vi "New from extension bytes.vi"(9 "Ext size":T1, 10 "Payload bytes":u8[](array[numeric]), 11 "Payload Ext Type":i8) -> (0 "error out":errorcluster, 3 "MsgPackExt out":refnum<class "MsgPackExt.lvclass">)   [LabVIEW 2020, in "MessagePack.lvlib" / "MsgPackExt.lvclass"]
uses:
  MsgPackExt.lvclass
  Requested ext size.ctl
  Typedefs/MsgPack Object Types.ctl
  MsgPackExt.lvclass/MsgPackExt.ctl
  MessagePack.lvlib
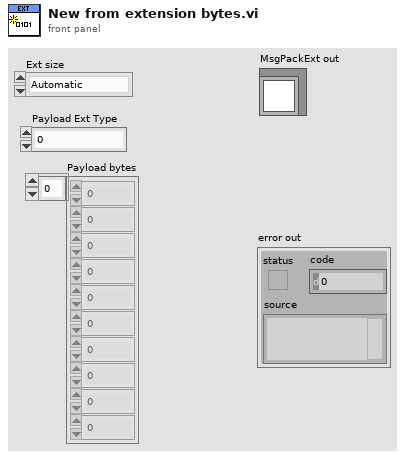
[diagram p1: front panel]
types:
  T1 = typedef "MessagePack.lvlib/MsgPackExt.lvclass/Requested ext size.ctl" = enum16{"Automatic", "Fixed 1-byte", "Fixed 2-bytes", "Fixed 4-bytes", "Fixed 8-bytes", "Fixed 16-bytes", "Up to 8 bytes", "Up to 16 bytes", "Up to 32 bytes"}
  T2 = typedef "MessagePack.lvlib/MsgPack Object Types.ctl" = enum16{"UNSUPPORTED", "POSINT", "NEGINT", "FIXMAP", "FIXARRAY", "FIXSTR", "NIL", "FALSE", "TRUE", "BIN8", "BIN16", "BIN32", "EXT8", "EXT16", "EXT32", "FLOAT32", "FLOAT64", "UINT8", "UINT16", "UINT32", "UINT64", "INT8", "INT16", "INT32", "INT64", "FIXEXT1", "FIXEXT2", "FIXEXT4", "FIXEXT8", "FIXEXT16", "STR8", "STR16", "STR32", "ARRAY16", "ARRAY32", "MAP16", "MAP32"}
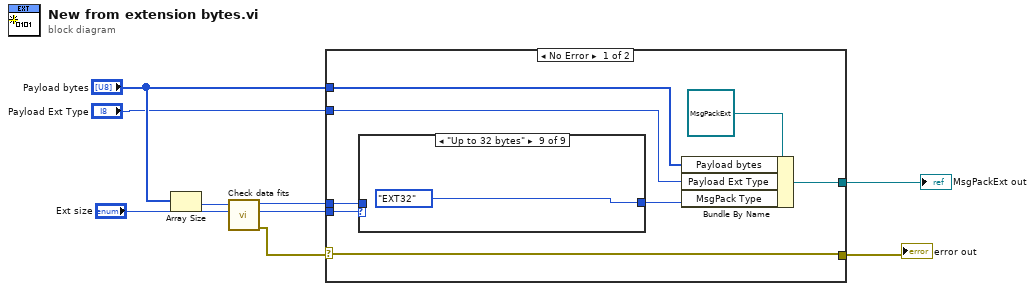
[diagram p0: block diagram]
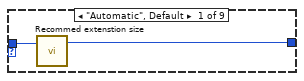
[diagram p2: hidden frame]
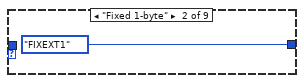
[diagram p3: hidden frame]
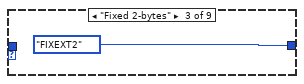
[diagram p4: hidden frame]
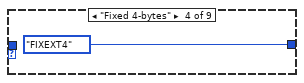
[diagram p5: hidden frame]
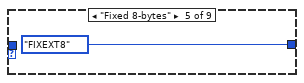
[diagram p6: hidden frame]
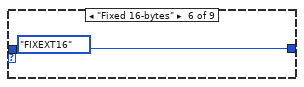
[diagram p7: hidden frame]
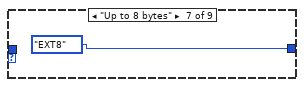
[diagram p8: hidden frame]
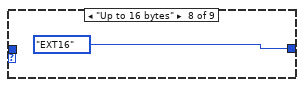
[diagram p9: hidden frame]
diagram:
  n1 = Array Size(array="Payload bytes") -> (size(s)=w7:i32)
  n2 = call "Check data fits.vi"("Ext size"="Ext size", "size"=w7) -> ("error out"=w1:errorcluster, "Ext size"=w4:T1, "size"=w5:u32)  [unwired: 7 in]
  n3 = case shown="No Error" w1 {
    selector: w1 -> [w12 w28]
    tunnel: [w16 _] -> w9
    tunnel: [w12 w28] -> w8
    tunnel: w5 -> [w15 _]
    tunnel: w4 -> [w14 _]
    tunnel: "Payload bytes" -> [w13 _]
    tunnel: "Payload Ext Type" -> [w11 _]
    frame No Error {
      n4 = case shown="\"Up to 32 bytes\"" w14 {
        tunnel: [w19 MsgPack_Object_Types."FIXEXT1" ("MsgPack Type") MsgPack_Object_Types."FIXEXT2" ("MsgPack Type") MsgPack_Object_Types."FIXEXT4" ("MsgPack Type") MsgPack_Object_Types."FIXEXT8" ("MsgPack Type") MsgPack_Object_Types."FIXEXT16" ("MsgPack Type") MsgPack_Object_Types."EXT8" ("MsgPack Type") MsgPack_Object_Types."EXT16" ("MsgPack Type") MsgPack_Object_Types."EXT32" ("MsgPack Type")] -> w10
        tunnel: w15 -> [w18 _ _ _ _ _ _ _ _]
        frame "Automatic", Default {
          n5 = call "Recommed extenstion size.vi"("size"=w18) -> ("MsgPack Type"=w19:T2)  [unwired: 2 in]
        }
        frame "Fixed 1-byte" {
        }
        frame "Fixed 2-bytes" {
        }
        frame "Fixed 4-bytes" {
        }
        frame "Fixed 8-bytes" {
        }
        frame "Fixed 16-bytes" {
        }
        frame "Up to 8 bytes" {
        }
        frame "Up to 16 bytes" {
        }
        frame "Up to 32 bytes" {
        }
      }
      n6 = Bundle By Name(cluster=refnum<class "MsgPackExt.lvclass"> refnum ("MessagePack.lvlib:MsgPackExt.lvclass"), "Payload bytes"=w13, "Payload Ext Type"=w11, "MsgPack Type"=w10) -> (w16:refnum<class "MsgPackExt.lvclass">)
    }
    frame Error {
    }
  }
  "error out" <- w8
  "MsgPackExt out" <- w9
